vi "Read Attributes.vi"(11 "Status Updated Msg":refnum<class "Status Updated Msg.lvclass">) -> (2 "Payload":cluster{"Status":string})   [LabVIEW 2020, in "Chat Window UI Controller.lvlib" / "Status Updated Msg.lvclass"]
uses:
  Status Updated Msg.lvclass
  Status Updated Msg.lvclass/Status Updated Msg.ctl
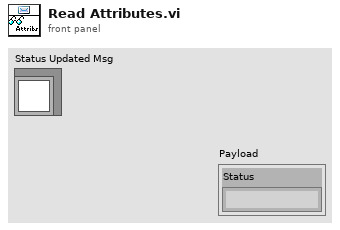
[diagram p1: front panel]
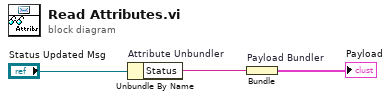
[diagram p0: block diagram]
diagram:
  n1 = Unbundle By Name "Attribute Unbundler"("Status Updated Msg") -> ("Status"=w1:string)
  n2 = Bundle "Payload Bundler"("Status"=w1) -> (→"Payload":cluster{"Status":string})  [unwired: 1 in]
